vi "VsEP I-O Controller.vi"(11 "Expt State (in)":T1={"Experimenter"="XYZ", "Number"=999, "Right"="Right", "Left"="Left", "Data Folder"=path "C:/Data/XYZ DATA/XYZ999", "State File"=path "C:/Data/XYZ DATA/XYZ999/Experiment State.txt", "Version Info"="CFTS VIs: V1.0 (190)\nExperiment VIs: 169\nLabVIEW.exe: V9.0f2 (2009)\nDAQmx: V9.0", "End Exposure Time"=-1.0, "Exposure Duration"="", "Run #"={"CAP"=0, "ABR"=12, "DP"=4, "VsEP"=0, "MeasSeq"=58, "SubSeq"=0, "SFOAE"=0}}) -> (3 "state out":T1)   [LabVIEW 2020]
uses:
  epl-vi-lib/Utility VIs/Buttons/KCheckmarkBoolean 2.ctl
  Typedefs/VsEP-Stimulus Control.ctl
  Typedefs/VsEP-Hidden Params.ctl
  epl-vi-lib/Signal Synthesis VIs/Controls/Gate XCtl/Gate Control.xctl
  CFTS Main Panel SubVIs/CFTS-Experiment State.ctl
  Typedefs/VsEP-Analysis State.ctl
  Typedefs/VsEP-Parameters.ctl
  CFTS Main Panel SubVIs/CFTS-Data Type Enum.ctl
panel:
  out "Atten (dB)":dbl
  in  "Params":T2={"STIMULUS"={"START dB re 1g/ms"=-6, "STOP dB re 1g/ms"=6, "dB STEPSIZE"=3.0, "REP RATE (/sec)"=17.0, "Alternate Polarity"=TRUE, "Sampling Rate (Hz)"=0.0}, "RESPONSE"={"Grass Gain"=10000, "#AVERAGES"=512, "Time Window (ms)"=20.0, "Fast Steps Threshold"=0}, "Hidden"={"AO Sampling Rate (Hz)"=100000.0, "AI Sampling Rate (Hz)"=100000.0, "Masker Timing"={"Active"=FALSE, "Delay (ms)"=0.0, "Width (ms)"=0.0, "Ramp (ms)"=0.0}, "Jerk rise time (ms)"=2.0, "Masker atten"=0.0, "show adjust"=FALSE, "linear gain"=FALSE}} {"STIMULUS"."dB STEPSIZE" format="%#_3g"; "STIMULUS"."START dB re 1g/ms" step=5}
  out "finished":T5={"path"=path "C:/Data/XYZ DATA/XYZ999/VsEP-999-2", "state"={"Experimenter"="XYZ", "Number"=999, "Right"="Right", "Left"="Left", "Data Folder"=path "C:/Data/XYZ DATA/XYZ999", "State File"=path "C:/Data/XYZ DATA/XYZ999/Experiment State.txt", "Version Info"="CFTS VIs: V1.0 (190)\nExperiment VIs: 169\nLabVIEW.exe: V9.0f2 (2009)\nDAQmx: V9.0", "End Exposure Time"=-1.0, "Exposure Duration"="", "Run #"={"CAP"=0, "ABR"=12, "DP"=4, "VsEP"=0, "MeasSeq"=58, "SubSeq"=0, "SFOAE"=0}}, "error"={"status"=FALSE, "code"=0, "source"=""}}
  in  "Analysis":T6
  out "MAX":dbl format="%.2f"
  out "Level":dbl=9.0
  out "User":string="XYZ"
  out "Run #":u16=2
  out "ID #":u16=999
  in  "Hidden":T4={"AO Sampling Rate (Hz)"=100000.0, "AI Sampling Rate (Hz)"=100000.0, "Masker Timing"={"Active"=FALSE, "Delay (ms)"=4.0, "Width (ms)"=0.0, "Ramp (ms)"=1.0}, "Jerk rise time (ms)"=2.0, "Masker atten"=0.0, "show adjust"=FALSE, "linear gain"=FALSE}
  in  "RESPONSE":T7={"Grass Gain"=10000, "#AVERAGES"=512, "Time Window (ms)"=8.5, "Fast Steps Threshold"=10000} {"Time Window (ms)" format="%.2f"}
  in  "STIMULUS":T3={"START dB re 1g/ms"=-15, "STOP dB re 1g/ms"=10, "dB STEPSIZE"=2.5, "REP RATE (/sec)"=17.0, "Alternate Polarity"=FALSE, "Sampling Rate (Hz)"=0.0} {"dB STEPSIZE" format="%#_3g"; "START dB re 1g/ms" step=5}
  out "Datafile path":path=path "C:/Data/XYZ DATA/XYZ999/VsEP-999-2"
  in  "Normalize traces":T8 caption="Normalize individual traces"
  in  "START":bool
  in  "RETURN":bool
  in  "STOP":bool
  out "Abort":bool
  out "CM":cluster{i32, dbl, dbl[][]}(graph)={0, 0.01, []} caption="\"Haircell component\""
  out "Neural":cluster{i32, dbl, dbl[][]}(graph)={0, 0.01, []}
  out "I-O":cluster{ext[], ext[]}[](graph)
  in  "NOTES":string
  # "Stimulus"
  # "Response"
  # "Running Average"
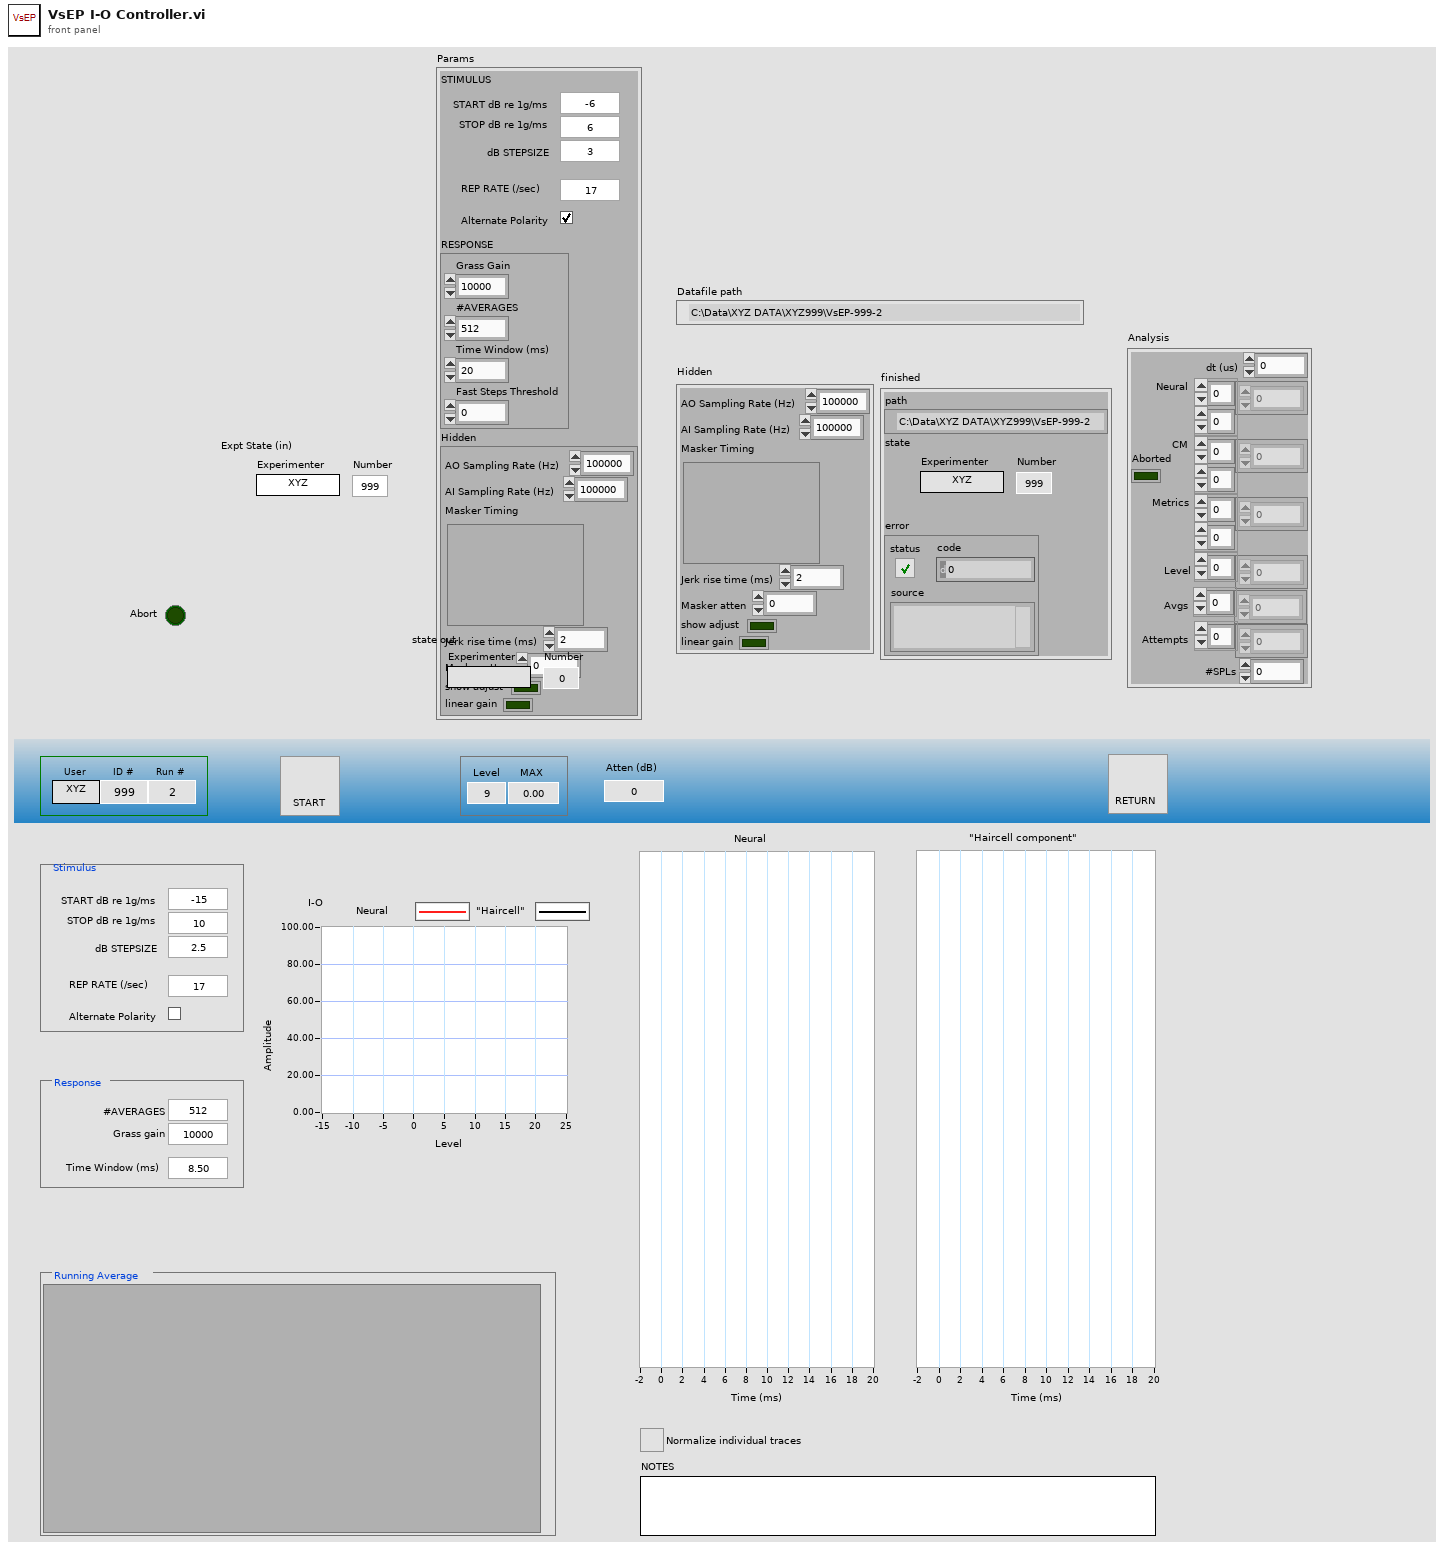
[diagram p1: front panel]
types:
  T1 = typedef "CFTS-Experiment State.ctl" = cluster{"Experimenter":string, "Number":u32, "Right":string, "Left":string, "Data Folder":path, "State File":path, "Version Info":string, "End Exposure Time":dbl, "Exposure Duration":string, "Run #":cluster{"CAP":i16, "ABR":i16, "DP":i16, "VsEP":i16, "MeasSeq":i16, "SubSeq":i16, "SFOAE":i16}}
  T2 = typedef "VsEP-Parameters.ctl" = cluster{"STIMULUS":T3, "RESPONSE":cluster{"Grass Gain":i32, "#AVERAGES":i32, "Time Window (ms)":sgl, "Fast Steps Threshold":i32}, "Hidden":T4}
  T3 = typedef "VsEP-Stimulus Control.ctl" = cluster{"START dB re 1g/ms":i32, "STOP dB re 1g/ms":i32, "dB STEPSIZE":sgl, "REP RATE (/sec)":dbl, "Alternate Polarity":bool, "Sampling Rate (Hz)":dbl}
  T4 = typedef "VsEP-Hidden Params.ctl" = cluster{"AO Sampling Rate (Hz)":dbl, "AI Sampling Rate (Hz)":dbl, "Masker Timing":cluster{"Active":bool, "Delay (ms)":dbl, "Width (ms)":dbl, "Ramp (ms)":dbl}, "Jerk rise time (ms)":dbl, "Masker atten":dbl, "show adjust":bool, "linear gain":bool}
  T5 = cluster{"path":path, "state":T1, "error":errorcluster}
  T6 = typedef "VsEP-Analysis State.ctl" = cluster{"dt (us)":dbl, "Neural":dbl[][], "CM":dbl[][], "Metrics":dbl[][], "Level":dbl[], "Avgs":i32[], "Attempts":i32[], "Aborted":bool, "#SPLs":i32}
  T7 = cluster{"Grass Gain":i32, "#AVERAGES":i32, "Time Window (ms)":sgl, "Fast Steps Threshold":i32}
  T8 = typedef "KCheckmarkBoolean 2.ctl" = bool
  T9 = cluster{"Neural":refnum<vi>, "CM":refnum<vi>, "I-O":refnum<vi>}
  T10 = cluster{"STIMULUS":T3, "RESPONSE":cluster{"Grass Gain":i32, "#AVERAGES":i32, "Time Window (ms)":sgl, "Fast Steps Threshold":i32}, "Hidden":T4}
  T11 = cluster{cluster{"STIMULUS":T3, "RESPONSE":cluster{"Grass Gain":i32, "#AVERAGES":i32, "Time Window (ms)":sgl, "Fast Steps Threshold":i32}, "Hidden":T4}, "state":T1}
  T12 = typedef "CFTS-Data Type Enum.ctl" = enum16{"CAP", "ABR", "DP", "VsEP", "MeasSeq", "SFOAE"}
  T13 = typedef "VsEP-Runtime Data.ctl" = cluster{"chan":i32[], "Ceiling":dbl, "dt (us)":dbl, "Crossed?":bool, "Step":dbl, "Stop":i32, "Avgs":i32, "Level":dbl, "AI Npts":i32, "Doubled?":bool, "reps/frame":i32, "altpol":bool, "AO npts":i32, "win Npts":i32, "gain":dbl}
  T14 = cluster{"Datafile path":path, "Expt State out":T1, "error out":errorcluster}
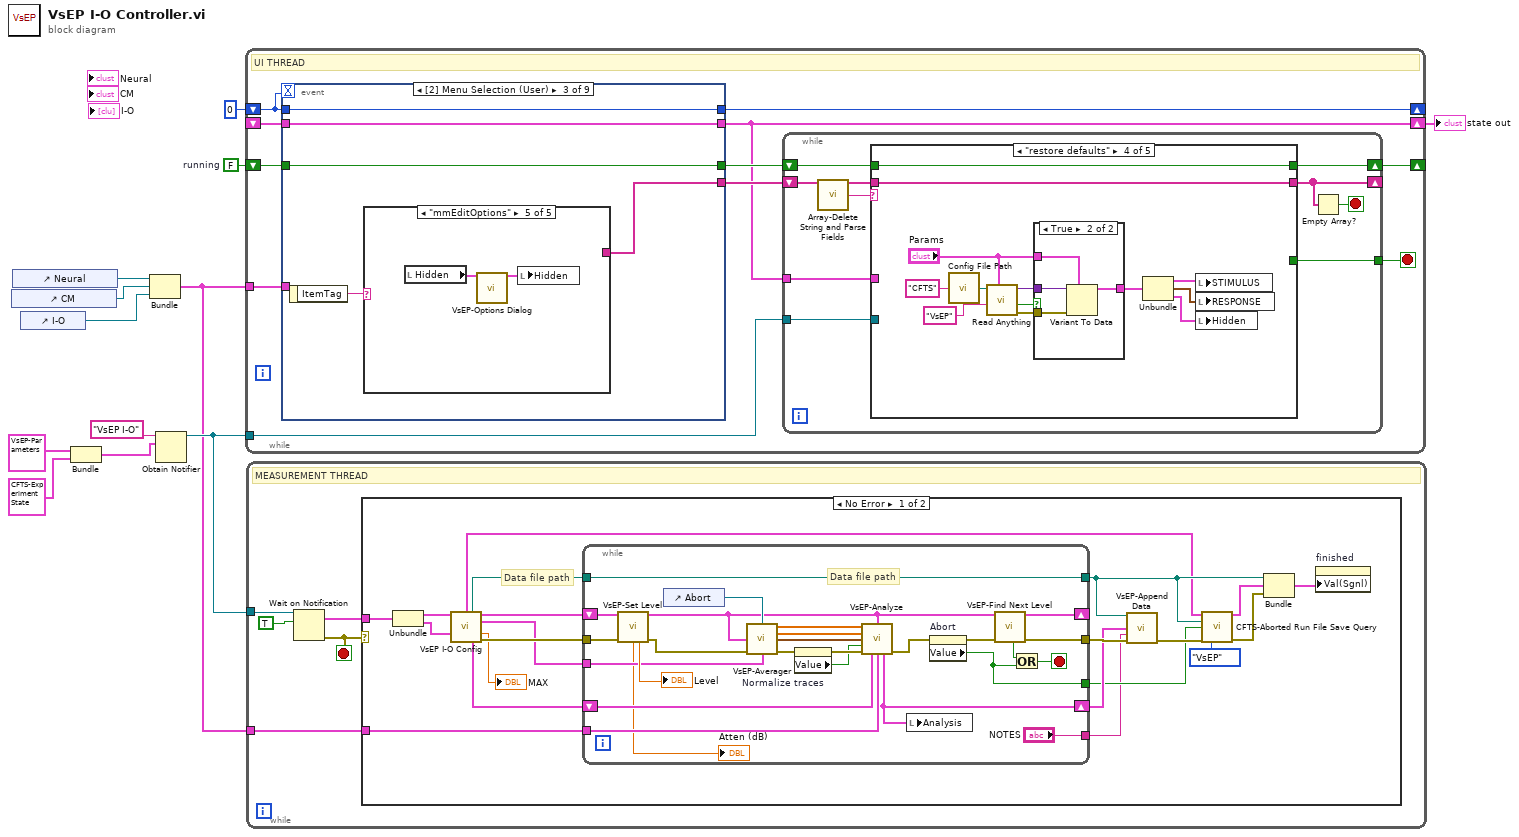
[diagram p0: block diagram]
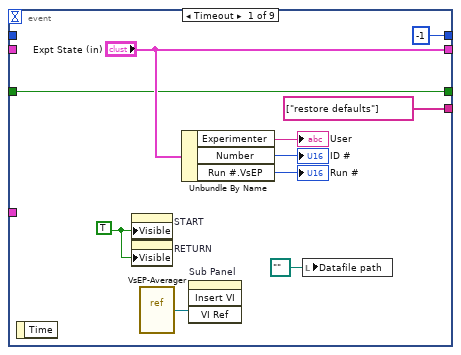
[diagram p2: hidden frame]
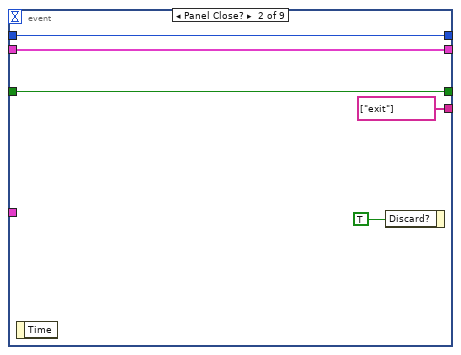
[diagram p3: hidden frame]
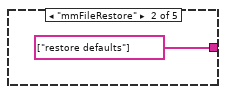
[diagram p5: hidden frame]
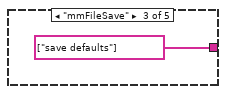
[diagram p6: hidden frame]
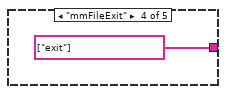
[diagram p7: hidden frame]
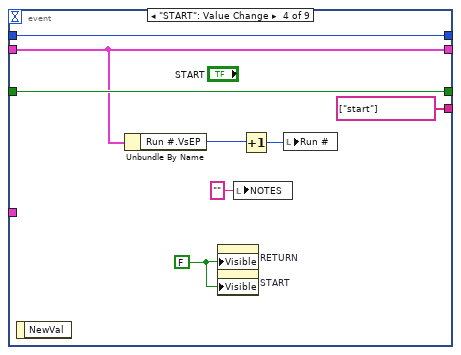
[diagram p8: hidden frame]
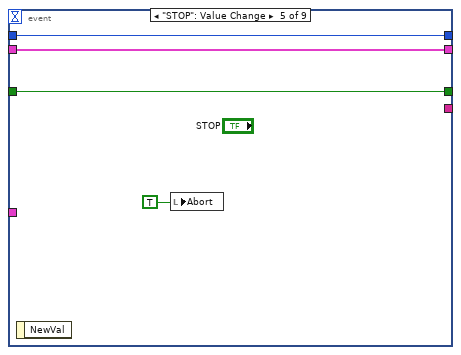
[diagram p9: hidden frame]
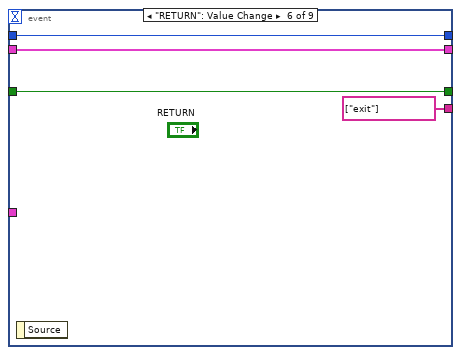
[diagram p10: hidden frame]
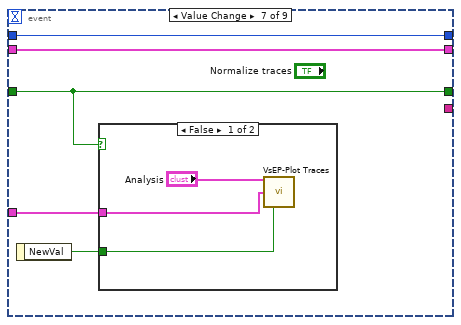
[diagram p11: hidden frame]
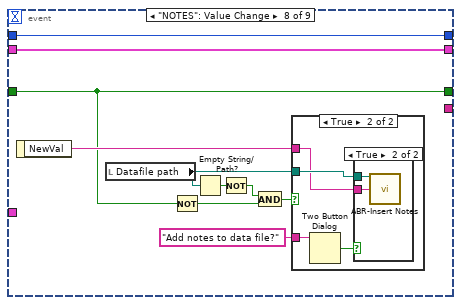
[diagram p13: hidden frame]
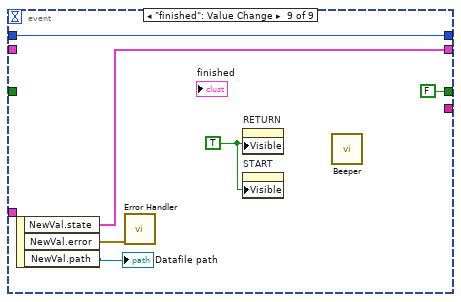
[diagram p16: hidden frame]
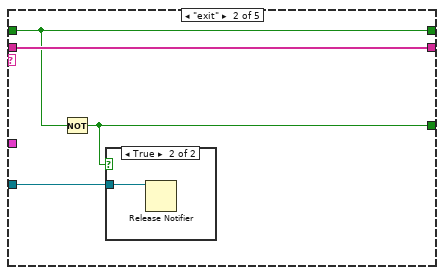
[diagram p18: hidden frame]
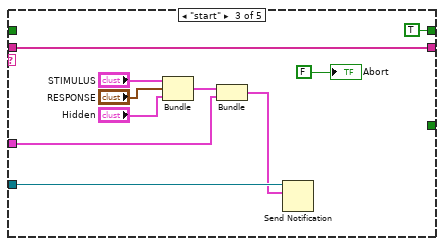
[diagram p20: hidden frame]
diagram:
  w2 = FALSE  # running
  n1 = control-ref of="CM"() -> (w8:refnum<vi>)
  n2 = control-ref of="Neural"() -> (w7:refnum<vi>)
  n3 = control-ref of="I-O"() -> (w9:refnum<vi>)
  n4 = Bundle("Params"=T2 {"STIMULUS"={"START dB re 1g/ms"=0, "STOP dB re 1g/ms"=0, "dB STEPSIZE"=0.0, "REP RATE (/sec)"=0.0, "Alternate Polarity"=FALSE, "Sampling Rate (Hz)"=0.0}, "RESPONSE"={"Grass Gain"=0, "#AVERAGES"=0, "Time Window (ms)"=0.0, "Fast Steps Threshold"=0}, "Hidden"={"AO Sampling Rate (Hz)"=0.0, "AI Sampling Rate (Hz)"=0.0, "Masker Timing"={"Active"=FALSE, "Delay (ms)"=0.0, "Width (ms)"=0.0, "Ramp (ms)"=0.0}, "Jerk rise time (ms)"=0.0, "Masker atten"=0.0, "show adjust"=FALSE, "linear gain"=FALSE}}, "Expt State (in) 2"=T1 {"Experimenter"="XYZ", "Number"=999, "Right"="Right", "Left"="Left", "Data Folder"=path "C:/Data/XYZ DATA/XYZ999", "State File"=path "C:/Data/XYZ DATA/XYZ999/Experiment State.txt", "Version Info"="CFTS VIs: V1.0 (190)\nExperiment VIs: 169\nLabVIEW.exe: V9.0f2 (2009)\nDAQmx: V9.0", "End Exposure Time"=-1.0, "Exposure Duration"="", "Run #"={"CAP"=0, "ABR"=12, "DP"=4, "VsEP"=0, "MeasSeq"=58, "SubSeq"=0, "SFOAE"=0}}) -> (w3:cluster{"Params":T2, "Expt State (in) 2":T1})  [unwired: 1 in]
  n5 = Bundle("Neural"=w7, "CM"=w8, "I-O"=w9) -> (w6:T9)  [unwired: 1 in]
  n6 = Obtain Notifier(name (unnamed)="VsEP I-O", notification data type=w3) -> (notifier out=w12:refnum<notifier>)  [unwired: 2 in, 2 out]
  n7 = while {
    tunnel: w12 -> [w17]
    shift-right: [w23] -> _
    shift-left: 0 -> [w22]
    tunnel: w6 -> [w21]
    shift-right: [w13] -> w1
    shift-left: _ -> [w20]
    shift-right: [w14] -> _
    shift-left: w2 -> [w15]
    stop <- w18 stop-if-true
    # "UI THREAD"
    n8 = event shown="[2] Menu Selection (User)" {
      selector: _ -> [_ _ _ _ _ _ _ _ _]
      dyn-events: _ -> [_ _ _ _ _ _ _ _ _]
      timeout: w22 -> [_ _ _ _ _ _ _ _ _]
      tunnel: [-1 w37 w43 w52 w59 w64 w67 w75 w92] -> w23
      tunnel: w22 -> [_ w37 w43 w52 w59 w64 w67 w75 w92]
      tunnel: w21 -> [_ _ _ _ _ _ w68 _ _]
      tunnel: ["Expt State (in)" w36 w42 w50 w58 w63 w66 w74 w90] -> w13
      tunnel: w20 -> [_ w36 w42 w50 w58 w63 w66 w74 _]
      tunnel: [string[] ["restore defaults"] string[] ["exit"] w39 string[] ["start"] _ string[] ["exit"] _ _ _] -> w19
      tunnel: [w24 w35 w41 w51 w57 w62 w65 w73 FALSE ("running")] -> w16
      tunnel: w15 -> [w24 w35 w41 w51 w57 w62 w65 w73 _]
      event Timeout {
        w29 = TRUE
        n9 = event-data() -> ()  [unwired: 1 in, 1 out]
        n10 = property on="START" class="Bool"("Visible"=w29) -> ()  [unwired: 2 in, 2 out]
        n11 = property on="RETURN" class="Bool"("Visible"=w29) -> ()  [unwired: 2 in, 2 out]
        n12 = vi-ref "VsEP-Averager.vi"() -> (w32:refnum<vi>)
        n13 = Unbundle By Name("Expt State (in)") -> ("Experimenter"=→"User":string, "Number"=→"ID #":u32, "Run #.VsEP"=→"Run #":i16)
        n14 = invoke on="Sub Panel" class="SubPanel" method="Insert VI"("VI Ref"=w32) -> ()  [unwired: 3 in, 4 out]
        n15 = local write "Datafile path"(path "" ("Datafile path")) -> ()
      }
      event Panel Close? {
        n16 = event-data() -> ()  [unwired: 1 in, 1 out]
        n17 = event-data("Discard?"=TRUE) -> ()  [unwired: 1 in, 1 out]
      }
      event Menu Selection (User) {
        n18 = event-data() -> ("ItemTag"=w40:string)  [unwired: 1 in]
        n19 = case shown="\"mmEditOptions\"" w40 {
          tunnel: [_ string[] ["restore defaults"] string[] ["save defaults"] string[] ["exit"] _] -> w39
          frame "False", Default {
          }
          frame "mmFileRestore" {
          }
          frame "mmFileSave" {
          }
          frame "mmFileExit" {
          }
          frame "mmEditOptions" {
            n20 = local read "Hidden"() -> (w48:T4)
            n21 = call "VsEP-Options Dialog.vi"("Options In"=w48) -> ("Options OUt"=w47:T4)  [unwired: 13 in, 1 out]
            n22 = local write "Hidden"(w47) -> ()
          }
        }
      }
      event "START": Value Change {
        w54 = FALSE ("ABI Abort")
        n23 = event-data() -> ()  [unwired: 1 in, 1 out]
        n24 = Unbundle By Name(w50) -> ("Run #.VsEP"=w56:i16)
        n25 = property on="RETURN" class="Bool"("Visible"=w54) -> ()  [unwired: 2 in, 2 out]
        n26 = property on="START" class="Bool"("Visible"=w54) -> ()  [unwired: 2 in, 2 out]
        n27 = local write "NOTES"("" ("NOTES")) -> ()
        n28 = Increment(x=w56) -> (x+1=w55:i16)
        n29 = local write "Run #"(w55) -> ()
      }
      event "STOP": Value Change {
        n30 = event-data() -> ()  [unwired: 1 in, 1 out]
        n31 = local write "Abort"(TRUE ("Stopping")) -> ()
      }
      event "RETURN": Value Change {
        n32 = event-data() -> ()  [unwired: 1 in, 1 out]
      }
      event Value Change {
        n33 = event-data() -> ("NewVal"=w69:T8)  [unwired: 1 in]
        n34 = case shown="False" w65 {
          tunnel: w69 -> [w70 _]
          tunnel: w68 -> [w71 _]
          frame False {
            n35 = call "VsEP-Plot Traces.vi"("Analysis"="Analysis", "Graphs"=w71, "Normalize individual?"=w70) -> ()  [unwired: 12 in, 1 out]
          }
          frame True {
          }
        }
      }
      event "NOTES": Value Change {
        n36 = event-data() -> ("NewVal"=w77:string)  [unwired: 1 in]
        n37 = local read "Datafile path"() -> (w78:path)
        n38 = Not(x=w73) -> (.not. x?=w81:bool)
        n39 = Empty String/Path?(string/path=w78) -> (empty?=w82:bool)
        n40 = Not(x=w82) -> (.not. x?=w80:bool)
        n41 = And(x=w80, y=w81) -> (x .and. y?=w79:bool)
        n42 = case shown="True" w79 {
          tunnel: w78 -> [_ w86]
          tunnel: w77 -> [_ w85]
          tunnel: "Add notes to data file?" ("message") -> [_ w84]
          frame False {
          }
          frame True {
            n43 = Two Button Dialog(message=w84) -> (T button?=w83:bool)  [unwired: 2 in]
            n44 = case shown="True" w83 {
              tunnel: w86 -> [_ w88]
              tunnel: w85 -> [_ w87]
              frame False {
              }
              frame True {
                n45 = call "ABR-Insert Notes.vi"("path"=w88, "Notes"=w87) -> ()  [unwired: 12 in, 2 out]
              }
            }
          }
        }
      }
      event "finished": Value Change {
        w94 = TRUE
        n46 = event-data() -> ("NewVal.state"=w90:T1, "NewVal.error"=w93:errorcluster, "NewVal.path"=→"Datafile path":path)  [unwired: 1 in]
        n47 = call "Error Handler.vi"("error in (no error)"=w93) -> ()  [unwired: 13 in, 2 out]
        n48 = property on="RETURN" class="Bool"("Visible"=w94) -> ()  [unwired: 2 in, 2 out]
        n49 = property on="START" class="Bool"("Visible"=w94) -> ()  [unwired: 2 in, 2 out]
        n50 = call "Beeper.vi"() -> ()  [unwired: 5 in, 1 out]
      }
    }
    n51 = while {
      shift-right: [w104] -> _
      shift-left: w19 -> [w101]
      tunnel: [w102] -> w18
      tunnel: w17 -> [w98]
      shift-right: [w96] -> w14
      shift-left: w16 -> [w97]
      tunnel: w13 -> [w95]
      stop <- w103 stop-if-true
      n52 = call "Array-Delete String and Parse Fields.vi"("Array in"=w101) -> ("Array out"=w100:string[], "Field 1"=w99:string)  [unwired: 10 in, 3 out]
      n53 = case shown="\"restore defaults\"" w99 {
        tunnel: w100 -> [w106 w110 w121 w134 w149]
        tunnel: [w106 w110 w121 w134 w149] -> w104
        tunnel: [_ w107 _ _ _] -> w102
        tunnel: w98 -> [_ w109 w116 _ _]
        tunnel: w97 -> [w105 w108 _ w133 _]
        tunnel: [w105 w108 TRUE ("running") w133 TRUE ("running")] -> w96
        tunnel: w95 -> [_ _ w117 _ _]
        frame "", Default {
        }
        frame "exit" {
          n54 = Not(x=w108) -> (.not. x?=w107:bool)
          n55 = case shown="True" w107 {
            tunnel: w109 -> [_ w111]
            frame False {
            }
            frame True {
              n56 = Release Notifier(notifier=w111) -> ()  [unwired: 2 in, 3 out]
            }
          }
        }
        frame "start" {
          n57 = Bundle("STIMULUS"="STIMULUS", "RESPONSE"="RESPONSE", "Hidden"="Hidden") -> (w118:T10)  [unwired: 1 in]
          n58 = Bundle(w118, "state"=w117) -> (w115:T11)  [unwired: 1 in]
          n59 = Send Notification(notification=w115, notifier=w116) -> ()  [unwired: 1 in, 2 out]
          "Abort" <- FALSE ("quitting")
        }
        frame "restore defaults" {
          n60 = call "Config File Path.vi"("AppName"="CFTS") -> ("Default config file name"=w131:path)
          n61 = call "Read Anything.vi"("Type of Anything"="Params", "Section Name (Name of \"Type of Anything\")"="VsEP" ("Section Name (Name of \"Type of Anything\")"), "Path (dialog)"=w131) -> ("Error Out"=w128:errorcluster, "Found?"=w129:bool, "Anything"=w127:variant)  [unwired: 6 in]
          n62 = case shown="True" w129 {
            tunnel: w128 -> [_ w139]
            tunnel: w127 -> [_ w138]
            tunnel: "Params" -> [w135 w137]
            tunnel: [w135 w136] -> w125
            frame False {
            }
            frame True {
              n63 = Variant To Data(error in=w139, type=w137, Variant=w138) -> (data=w136:T2)  [unwired: 1 out]
            }
          }
          n64 = Unbundle(w125) -> ("STIMULUS"=w124:T3, "RESPONSE"=w123:T7, "Hidden"=w122:T4)
          n65 = local write "STIMULUS"(w124) -> ()
          n66 = local write "RESPONSE"(w123) -> ()
          n67 = local write "Hidden"(w122) -> ()
        }
        frame "save defaults" {
          n68 = local read "RESPONSE"() -> (w146:T7)
          n69 = local read "STIMULUS"() -> (w147:T3)
          n70 = local read "Hidden"() -> (w145:T4)
          n71 = Bundle("STIMULUS"=w147, "RESPONSE"=w146, "Hidden"=w145) -> (w140:T10)  [unwired: 1 in]
          n72 = call "Config File Path.vi"("AppName"="CFTS") -> ("Default config file name"=w143:path)
          n73 = call "Write Anything.vi"("Section Name (Name of \"Anything\")"="VsEP" ("Section Name (Name of \"Type of Anything\")"), "Anything"=w140, "Path (dialog)"=w143) -> ("Error Out"=w141:errorcluster)  [unwired: 7 in, 1 out]
          n74 = call "Error Handler.vi"("error in (no error)"=w141) -> ()  [unwired: 13 in, 2 out]
        }
      }
      n75 = Empty Array?(array=w104) -> (empty?=w103:bool)
    }
  }
  "state out" <- w1
  n76 = while {
    tunnel: w12 -> [w153]
    tunnel: w6 -> [w151]
    stop <- w152 stop-if-true
    # "MEASUREMENT THREAD"
    n77 = Wait on Notification(notifier=w153, ignore previous (F)=TRUE) -> (notification=w150:cluster{"Params":T2, "Expt State (in) 2":T1}, error out=w152:errorcluster)  [unwired: 2 in, 2 out]
    n78 = case shown="No Error" w152 {
      tunnel: w151 -> [w167 _]
      tunnel: w150 -> [w165 _]
      frame No Error {
        # "Data file path"
        n79 = Unbundle(w165) -> ("Params"=w163:T2, "Expt State (in) 2"=w164:T1)
        n80 = call "VsEP I-O Config.vi"("Params"=w163, "Expt State"=w164) -> ("Expt State out"=w156:T1, "Datafile path"=w174:path, "Runtime"=w173:T13, "hidden out"=w172:T4, "Max SPL"=→"MAX":dbl, "Analysis"=w158:T6, "error out"=w175:errorcluster)  [unwired: 7 in]
        n81 = while {
          tunnel: w174 -> [w201]
          tunnel: [w201] -> w162
          shift-right: [w192] -> _
          shift-left: w173 -> [w196]
          tunnel: w175 -> [w198]
          tunnel: [w193] -> w171
          tunnel: w172 -> [w189]
          shift-right: [w178] -> w170
          shift-left: w158 -> [w183]
          tunnel: w167 -> [w180]
          tunnel: ["NOTES"] -> w155
          tunnel: [w177] -> w166
          stop <- w190 stop-if-true
          # "Data file path"
          # "stepsize"
          # "max SPL"
          # "array of levels"
          # "current SPL"
          n82 = call "VsEP-Set Level.vi"("Runtime"=w196, "error in (no error)"=w198) -> ("Runtime out"=w184:T13, "atten"=→"Atten (dB)":dbl, "Level"=→"Level":dbl, "error out"=w197:errorcluster)  [unwired: 10 in]
          n83 = control-ref of="Abort"() -> (w200:refnum<vi>)
          n84 = call "VsEP-Averager.vi"("Abort"=w200, "Runtime"=w184, "error in (no error)"=w197, "Hidden"=w189) -> ("Neural (uV)"=w188:dbl[], "microphonic (uV)"=w187:dbl[], "averaging data"=w181:cluster{i32, i32}, "error out"=w199:errorcluster)  [unwired: 8 in]
          n85 = property on="Normalize traces" class="Bool (strict)"(error in=w199) -> (error out=w186:errorcluster, "Value"=w182:T8)  [unwired: 1 in, 1 out]
          n86 = call "VsEP-Analyze.vi"("Neural (uV)"=w188, "Runtime"=w184, "microphonic (uV)"=w187, "Averaging data"=w181, "Normalize individual?"=w182, "error in"=w186, "Analysis"=w183, "Graphs"=w180) -> ("Analysis out"=w178:T6, "error out"=w185:errorcluster)  [unwired: 6 in]
          n87 = local write "Analysis"(w178) -> ()
          n88 = property on="Abort" class="Bool (strict)"(error in=w185) -> (error out=w194:errorcluster, "Value"=w177:bool)  [unwired: 1 in, 1 out]
          n89 = call "VsEP-Find Next Level.vi"("Runtime"=w184, "error in (no error)"=w194) -> ("Runtime out"=w192:T13, "Finished"=w191:bool, "error out"=w193:errorcluster)  [unwired: 11 in]
          n90 = Or(x=w191, y=w177) -> (x .or. y?=w190:bool)
        }
        n91 = call "VsEP-Append Data.vi"("path"=w162, "Analysis"=w170, "Notes"=w155, "error in (no error)"=w171) -> ("error out"=w169:errorcluster)  [unwired: 11 in]
        n92 = call "CFTS-Aborted Run File Save Query.vi"("Expt State"=w156, "Path"=w162, "Aborted"=w166, "error in (no error)"=w169, "Data Type"=CFTS-Data_Type_Enum."VsEP") -> ("Expt State out"=w161:T1, "error out"=w160:errorcluster)  [unwired: 8 in, 1 out]
        n93 = Bundle("Datafile path"=w162, "Expt State out"=w161, "error out"=w160) -> (w159:T14)  [unwired: 1 in]
        n94 = property on="finished" class="Clust (strict)"("Val(Sgnl)"=w159) -> ()  [unwired: 2 in, 2 out]
      }
      frame Error {
      }
    }
  }
